vi "condAmbientalesFinales.vi"(8 "error in (no error)":errorcluster, 11 "Calibrador in":refnum<class "Calibrador.lvclass">) -> (0 "error out":errorcluster, 3 "Calibrador out":refnum<class "Calibrador.lvclass">)   [LabVIEW 2019, in "Calibrador.lvclass"]
uses:
  Calibrador.lvclass
  Base de Datos/Base de Datos.lvclass
  Base de Datos/SQLiteConnector/SQLiteConnection.lvclass
panel:
  in  "salir":bool
  in  "presion":dbl
  out "presion_corregida":dbl
  out "presion_ok":bool
  in  "humedad":dbl
  out "humedad_corregida":dbl
  out "humedad_ok":bool
  in  "temperatura":dbl
  out "temp_corregida":dbl
  out "temp_ok":bool
  # "Medido"
  # "Corregido"
  # "Cumple"
  # "[°C]"
  # "[hPa]"
  # "[%]"
  # "Humedad"
  # "Presión"
  # "Temperatura"
  # "Condiciones Ambientales \nFINALES"
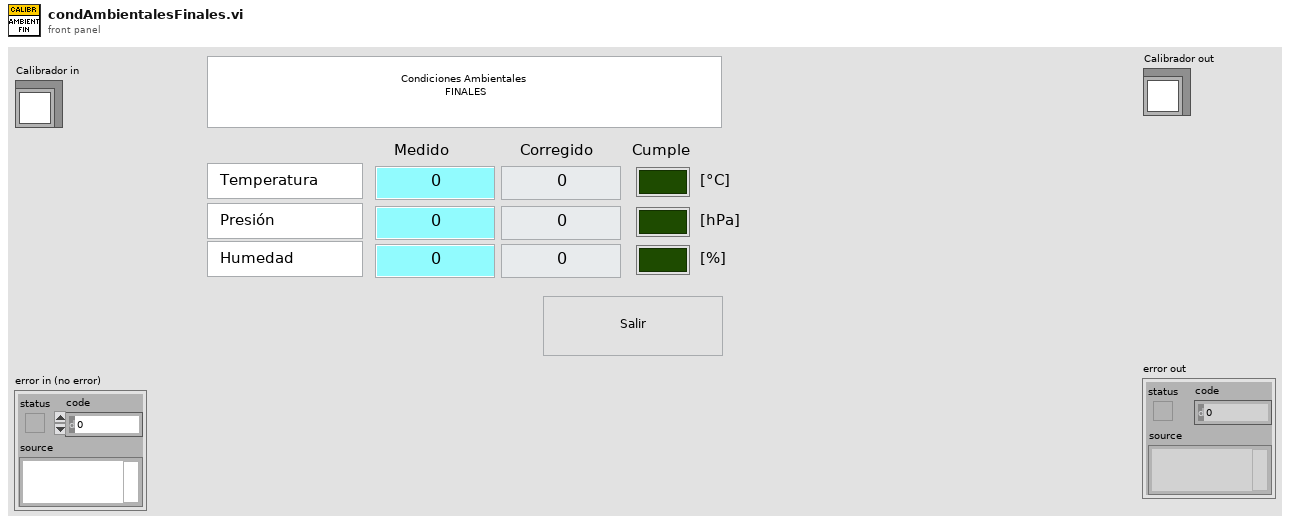
[diagram p1: front panel]
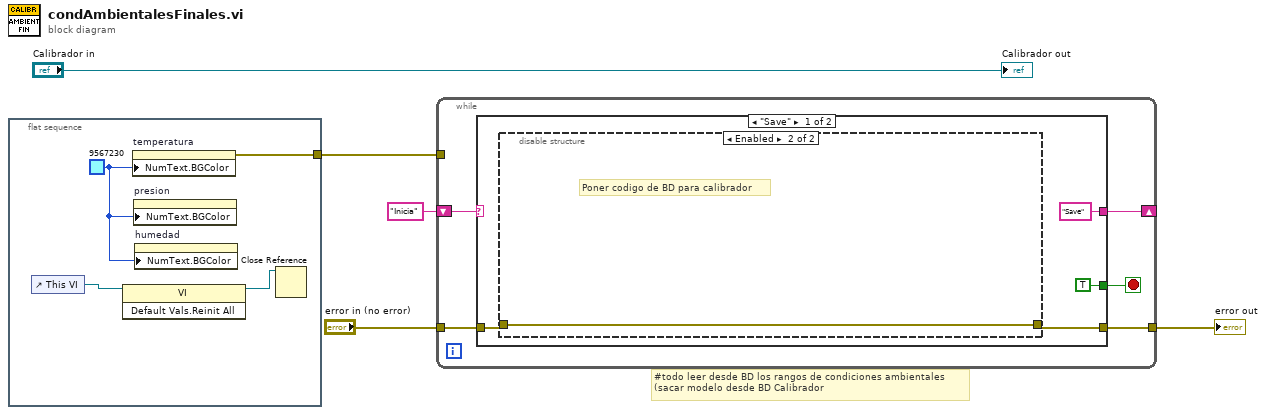
[diagram p0: block diagram]
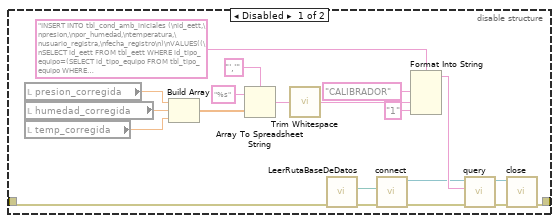
[diagram p2: hidden frame]
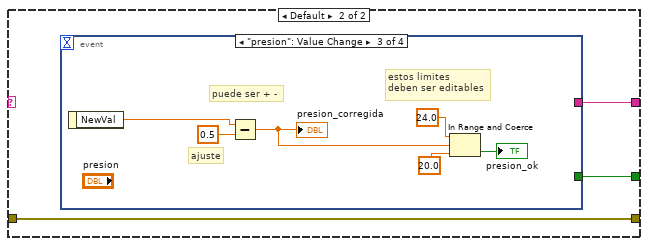
[diagram p3: hidden frame]
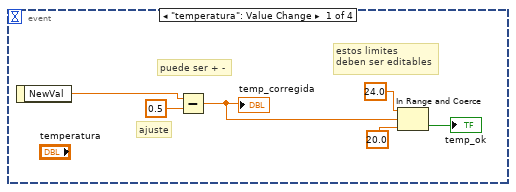
[diagram p4: hidden frame]
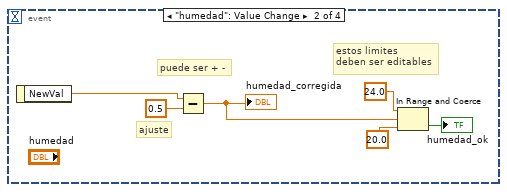
[diagram p5: hidden frame]
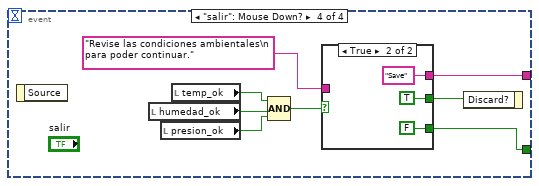
[diagram p6: hidden frame]
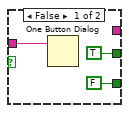
[diagram p7: hidden frame]
diagram:
  # "#todo leer desde BD los rangos de condiciones ambientales\n(sacar modelo desde BD Calibrador"
  n1 = flat-sequence {
    tunnel: [w8] -> w5
    frame #0 {
      w9 = u32 9567230
      n2 = control-ref of="This VI"() -> (w7:refnum<vi>)
      n3 = invoke class="VI" method="Default Vals.Reinit All"(reference=w7) -> (reference out=w6:refnum<vi>)  [unwired: 2 in, 2 out]
      n4 = property on="temperatura" class="DigNum (strict)"("NumText.BGColor"=w9) -> (error out=w8:errorcluster)  [unwired: 2 in, 1 out]
      n5 = property on="presion" class="DigNum (strict)"("NumText.BGColor"=w9) -> ()  [unwired: 2 in, 2 out]
      n6 = property on="humedad" class="DigNum (strict)"("NumText.BGColor"=w9) -> ()  [unwired: 2 in, 2 out]
      n7 = Close Reference(reference=w6) -> ()  [unwired: 1 in, 1 out]
    }
  }
  n8 = while {
    tunnel: w5 -> [_]
    shift-right: [w12] -> _
    shift-left: "Inicia" -> [w13]
    tunnel: "error in (no error)" -> [w11]
    tunnel: [w10] -> w1
    stop <- w14 stop-if-true
    n9 = case shown="\"Save\"" w13 {
      tunnel: [TRUE w42] -> w14
      tunnel: ["Save" w41] -> w12
      tunnel: w11 -> [w16 w40]
      tunnel: [w15 w40] -> w10
      frame "Save" {
        n10 = disable-structure shown="Enabled" {
          disable-tunnel: w16 -> [w20 w39]
          disable-tunnel: [w19 w39] -> w15
          frame Disabled {
            n11 = local read "presion_corregida"() -> (w22:dbl)
            n12 = local read "humedad_corregida"() -> (w23:dbl)
            n13 = local read "temp_corregida"() -> (w21:dbl)
            n14 = Build Array(w22, w23, w21) -> (w32:dbl[])
            n15 = Array To Spreadsheet String(delimiter (Tab)="','", array=w32, 3:"%s" ("format string")) -> (spreadsheet string=w36:string)
            n16 = call <vilib>:"Trim Whitespace.vi"("string"=w36) -> ("trimmed string"=w37:string)  [unwired: 1 in]
            n17 = call "LeerRutaBaseDeDatos.vi"("error in (no error)"=w20) -> ("error out"=w29:errorcluster, "Database Path"=w28:path)  [unwired: 9 in]
            n18 = call "connect.vi"("error in (no error)"=w29, "Database Path"=w28) -> ("error out"=w26:errorcluster, "object out"=w27:refnum<class "SQLiteConnection.lvclass">)  [unwired: 8 in]
            n19 = Format Into String(format string="INSERT INTO tbl_cond_amb_iniciales (\nid_eett,\npresion,\npor_humedad,\ntemperatura,\nusuario_registra,\nfecha_registro\n)\nVALUES((\nSELECT id_eett FROM tbl_eett WHERE id_tipo_equipo=(SELECT id_tipo_equipo FROM tbl_tipo_equipo WHERE nombre='%s')),'%s','%s',DATETIME('NOW'))" ("SQL Statement"), "CALIBRADOR" ("input 1"), w37, "1" ("input 2")) -> (resulting string=w31:string)  [unwired: 2 in, 1 out]
            n20 = call "query.vi"("error in (no error)"=w26, "SQL Statement"=w31, "object in"=w27) -> ("error out"=w24:errorcluster, "object out"=w25:refnum<class "SQLiteConnection.lvclass">)  [unwired: 5 in, 2 out]
            n21 = call-dynamic "close.vi"("error in (no error)"=w24, "object in"=w25) -> ("error out"=w19:errorcluster)  [unwired: 8 in, 1 out]
          }
          frame Enabled {
            # "Poner codigo de BD para calibrador"
          }
        }
      }
      frame Default {
        n22 = event shown="[2] \"presion\": Value Change" {
          selector: _ -> [_ _ _ _]
          dyn-events: _ -> [_ _ _ _]
          timeout: _ -> [_ _ _ _]
          tunnel: [_ _ _ w62] -> w42
          tunnel: [_ _ _ w61] -> w41
          event "temperatura": Value Change {
            # "estos limites\ndeben ser editables"
            # "puede ser + -"
            # "ajuste"
            n23 = event-data() -> ("NewVal"=w43:dbl)  [unwired: 1 in]
            n24 = Subtract(x=w43, y=0.5) -> (x-y=w48:dbl)
            "temp_corregida" <- w48
            n25 = In Range and Coerce(upper limit=24.0, x=w48, lower limit=20.0) -> (In Range?=→"temp_ok":bool)  [unwired: 1 out]
          }
          event "humedad": Value Change {
            # "estos limites\ndeben ser editables"
            # "puede ser + -"
            # "ajuste"
            n26 = event-data() -> ("NewVal"=w51:dbl)  [unwired: 1 in]
            n27 = Subtract(x=w51, y=0.5) -> (x-y=w50:dbl)
            "humedad_corregida" <- w50
            n28 = In Range and Coerce(upper limit=24.0, x=w50, lower limit=20.0) -> (In Range?=→"humedad_ok":bool)  [unwired: 1 out]
          }
          event "presion": Value Change {
            # "estos limites\ndeben ser editables"
            # "puede ser + -"
            # "ajuste"
            n29 = event-data() -> ("NewVal"=w57:dbl)  [unwired: 1 in]
            n30 = Subtract(x=w57, y=0.5) -> (x-y=w56:dbl)
            "presion_corregida" <- w56
            n31 = In Range and Coerce(upper limit=24.0, x=w56, lower limit=20.0) -> (In Range?=→"presion_ok":bool)  [unwired: 1 out]
          }
          event "salir": Mouse Down? {
            n32 = event-data() -> ()  [unwired: 1 in, 1 out]
            n33 = local read "humedad_ok"() -> (w67:bool)
            n34 = local read "presion_ok"() -> (w66:bool)
            n35 = local read "temp_ok"() -> (w68:bool)
            n36 = Compound Arithmetic op=AND(w68, w67, w66) -> (w65:bool)
            n37 = case shown="True" w65 {
              tunnel: "Revise las condiciones ambientales\n           para poder continuar." -> [w71 _]
              tunnel: [TRUE TRUE] -> w63
              tunnel: [FALSE FALSE] -> w62
              tunnel: [_ "Save"] -> w61
              frame False {
                n38 = One Button Dialog(message=w71) -> ()  [unwired: 1 in, 1 out]
              }
              frame True {
              }
            }
            n39 = event-data("Discard?"=w63) -> ()  [unwired: 1 in, 1 out]
          }
        }
      }
    }
  }
  "error out" <- w1
  "Calibrador out" <- "Calibrador in"
